vi "resetView.vi"(8 "error in (no error)":errorcluster, 11 "OutcomeListUIAdapter in":refnum<class "OutcomeListUIAdapter.lvclass">) -> (0 "error out":errorcluster, 3 "OutcomeListUIAdapter out":refnum<class "OutcomeListUIAdapter.lvclass">)   [LabVIEW 2018, in "OutcomeListUIAdapter.lvclass"]
uses:
  OutcomeListUIAdapter.lvclass
  <vilib>/Utility/miscctls.llb/LVRowAndColumnUnsignedTypeDef.ctl
  OutcomeListUIAdapter.lvclass/OutcomeListUIAdapter.ctl
  <vilib>/Utility/miscctls.llb/LVRowAndColumnTypeDef.ctl
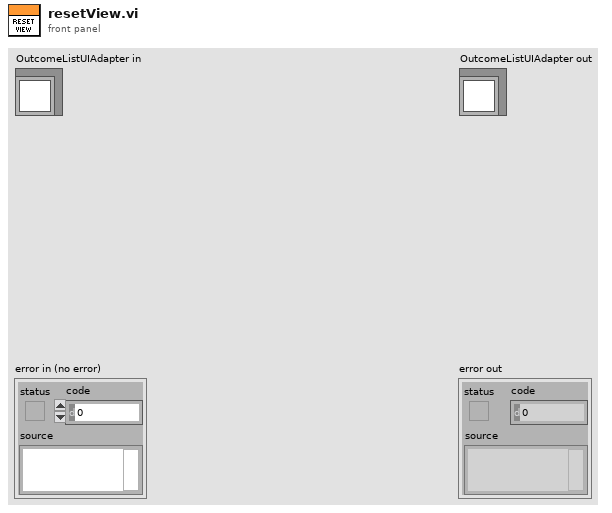
[diagram p1: front panel]
types:
  T1 = typedef "LVRowAndColumnUnsignedTypeDef.ctl" = cluster{"Row":u32, "Column":u32}
  T2 = typedef "LVRowAndColumnTypeDef.ctl" = cluster{"Row":i32, "Column":i32}
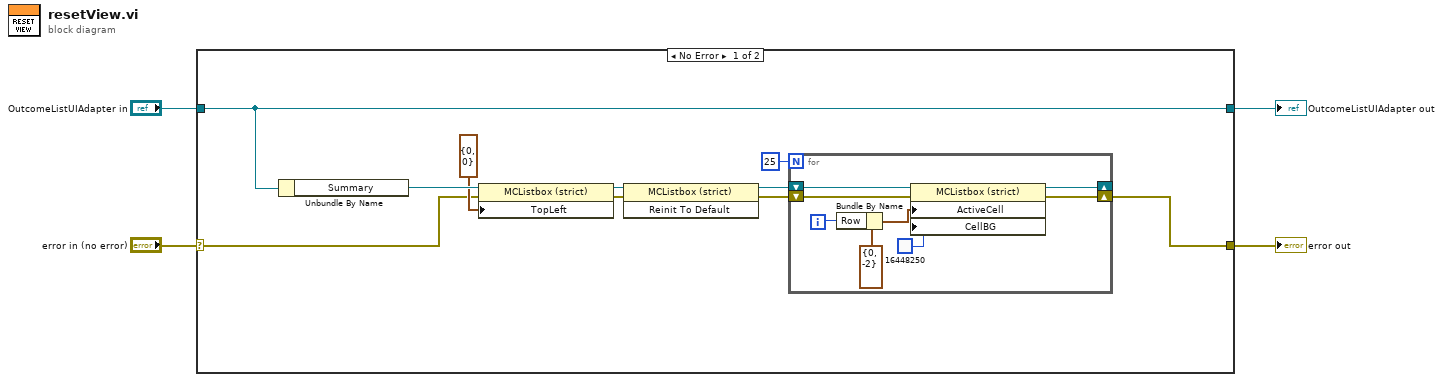
[diagram p0: block diagram]
diagram:
  n1 = case shown="No Error" "error in (no error)" {
    selector: "error in (no error)" -> [w6 w24]
    tunnel: [w5 w24] -> w3
    tunnel: [w7 w23] -> w1
    tunnel: "OutcomeListUIAdapter in" -> [w7 w23]
    frame No Error {
      n2 = Unbundle By Name(w7) -> ("Summary"=w14:refnum<vi>)
      n3 = property on="Property Node" class="MCListbox (strict)"(reference=w14, error in=w6, "TopLeft"=T1 {"Row"=0, "Column"=0} ("Top Left Visible Cell")) -> (reference out=w12:refnum<vi>, error out=w11:errorcluster)
      n4 = invoke class="MCListbox (strict)" method="Reinit To Default"(reference=w12, error in=w11) -> (reference out=w10:refnum<vi>, error out=w9:errorcluster)  [unwired: 1 in, 1 out]
      n5 = for {
        N: 25 -> [_]
        shift-right: [w21] -> _
        shift-left: w10 -> [w22]
        shift-right: [w19] -> w5
        shift-left: w9 -> [w20]
        i -> [w17]
        n6 = Bundle By Name(cluster=T2 {"Row"=0, "Column"=-2} ("Active Cell:Active Cell"), "Row"=w17) -> (w16:T2)
        n7 = property on="Property Node" class="MCListbox (strict)"(reference=w22, error in=w20, "ActiveCell"=w16, "CellBG"=u32 16448250) -> (reference out=w21:refnum<vi>, error out=w19:errorcluster)
      }
    }
    frame Error {
    }
  }
  "error out" <- w3
  "OutcomeListUIAdapter out" <- w1
